vi "Set Sensor Number.vi"(8 "error in (no error)":errorcluster, 10 "Sensor Number":i32, 11 "Project Number Msg in":refnum<class "Sensor Number Msg.lvclass">) -> (0 "error out":errorcluster, 3 "Project Number Msg out":refnum<class "Sensor Number Msg.lvclass">)   [LabVIEW 2013, in "Main Model.lvlib" / "Sensor Number Msg.lvclass"]
uses:
  Sensor Number Msg.lvclass
  Sensor Number Msg.lvclass/Sensor Number Msg.ctl
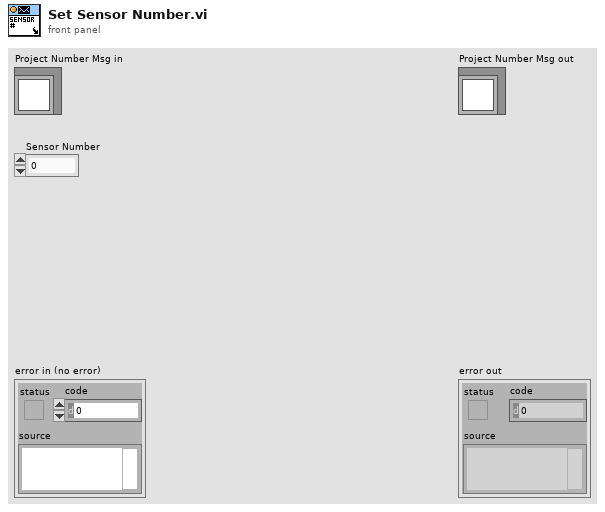
[diagram p1: front panel]
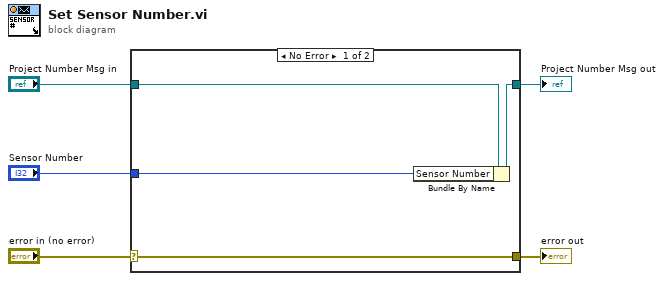
[diagram p0: block diagram]
diagram:
  n1 = case shown="No Error" "error in (no error)" {
    selector: "error in (no error)" -> [w9 w10]
    tunnel: [w9 w10] -> w4
    tunnel: [w7 w11] -> w2
    tunnel: "Project Number Msg in" -> [w8 w11]
    tunnel: "Sensor Number" -> [w6 _]
    frame No Error {
      n2 = Bundle By Name(cluster=w8, "Sensor Number"=w6) -> (w7:refnum<class "Sensor Number Msg.lvclass">)
    }
    frame Error {
    }
  }
  "error out" <- w4
  "Project Number Msg out" <- w2
